vi "SPI basic read write test.vi"() -> ()   [LabVIEW 2012]
uses:
  <vilib>/ni845x/ni845x.llb/ni845xControl.ctl
panel:
  out "read = write":bool
  in  "Stop":bool
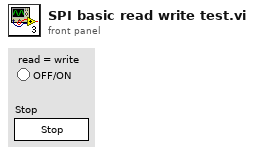
[diagram p1: front panel]
types:
  T1 = typedef "ni845xControl.ctl" = refnum<k21>
  T2 = typedef "AccelerometerSPI.ctl" = cluster{"Device":T1, "spi configuration":T3}
  T3 = typedef "ni845xSpiConfiguration.ctl" = refnum<k20>
  T4 = cluster{"device reference out":T1, "spi configuration out":T3}
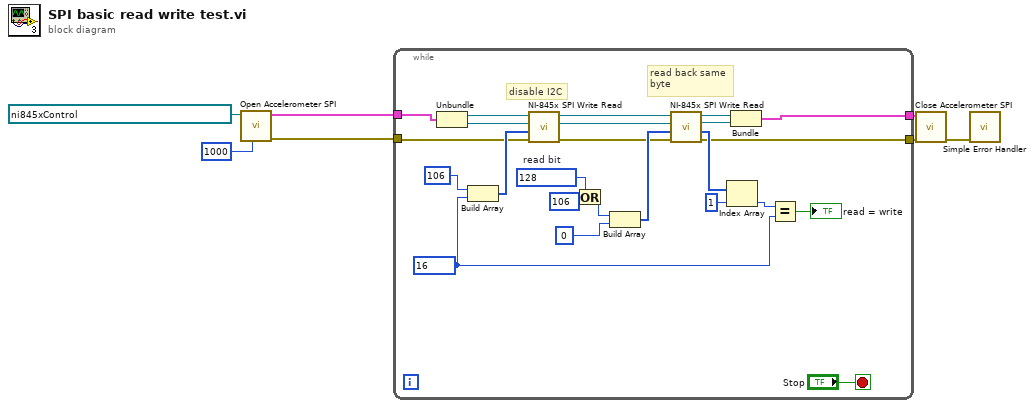
[diagram p0: block diagram]
diagram:
  n1 = call "Open Accelerometer SPI.vi"("Clock Rate in kHz"=u16 1000, "Device"=T1 "USB0::0x3923::0x7166::01879089::RAW") -> ("error out"=w3:errorcluster, "Accelerometer"=w4:T2)  [unwired: 8 in]
  n2 = while {
    tunnel: w4 -> [w26]
    tunnel: w3 -> [w25]
    tunnel: [w9] -> w2
    tunnel: [w8] -> w1
    stop <- "Stop" stop-if-true
    w17 = u8 128  # read bit
    w13 = u8 16
    # "read back same\nbyte"
    # "disable I2C"
    n3 = Unbundle(w26) -> ("Device"=w28:T1, "spi configuration"=w27:T3)
    n4 = Build Array(u8 106, w13) -> (w29:u8[])
    n5 = call <vilib>:"NI-845x SPI Write Read.vi"("error in (no error)"=w25, "write data"=w29, "spi configuration in"=w27, "device reference in"=w28) -> ("error out"=w19:errorcluster, "spi configuration out"=w20:T3, "device reference out"=w21:T1)  [unwired: 4 in, 1 out]
    n6 = Or(x=w17, y=u8 106) -> (x .or. y?=w18:u8)
    n7 = Build Array(w18, u8 0) -> (w24:u8[])
    n8 = call <vilib>:"NI-845x SPI Write Read.vi"("error in (no error)"=w19, "write data"=w24, "spi configuration in"=w20, "device reference in"=w21) -> ("error out"=w8:errorcluster, "read data"=w16:u8[], "spi configuration out"=w10:T3, "device reference out"=w11:T1)  [unwired: 4 in]
    n9 = Index Array(array=w16, index=1) -> (element=w14:u8)
    n10 = Bundle("device reference out"=w11, "spi configuration out"=w10) -> (w9:T4)  [unwired: 1 in]
    n11 = Equal?(x=w14, y=w13) -> (x = y?=→"read = write":bool)
  }
  n12 = call "Close Accelerometer SPI.vi"("error in (no error)"=w1, "Accelerometer"=w2) -> ("error out"=w5:errorcluster)  [unwired: 9 in]
  n13 = call <vilib>:"Simple Error Handler.vi"("error in (no error)"=w5) -> ()  [unwired: 4 in, 5 out]
